vi "popup_timer.vi"(1 "Seconds":dbl) -> (8 "Done":bool)   [LabVIEW 2016]
panel:
  in  "Time Display":bool
  out "Slide":u8(slide) scale=0.0..6.0
  # "Name"
  # "MVC Countdown"
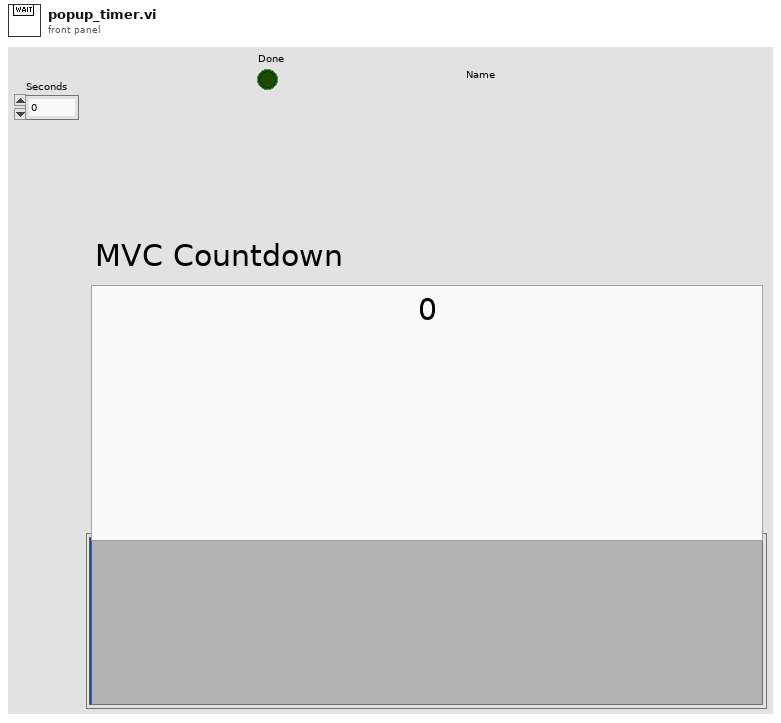
[diagram p1: front panel]
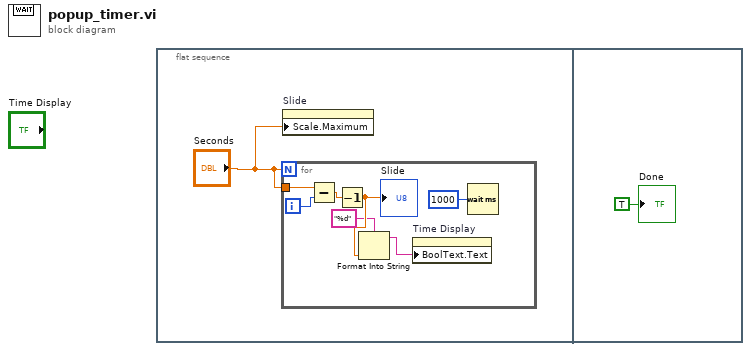
[diagram p0: block diagram]
diagram:
  n1 = flat-sequence {
    frame #0 {
      n2 = for {
        N: "Seconds" -> [_]
        tunnel: "Seconds" -> [w7]
        i -> [w6]
        n3 = Subtract(x=w7, y=w6) -> (x-y=w5:dbl)
        n4 = Decrement(x=w5) -> (x-1=w4:dbl)
        "Slide" <- w4
        n5 = Format Into String(format string="%d", w4) -> (resulting string=w3:string)  [unwired: 2 in, 1 out]
        n6 = property on="Time Display" class="Bool"("BoolText.Text"=w3) -> ()  [unwired: 2 in, 2 out]
        n7 = Wait (ms)(milliseconds to wait=u32 1000) -> ()  [unwired: 1 out]
      }
      n8 = property on="Slide" class="Slide (strict)"("Scale.Maximum"="Seconds") -> ()  [unwired: 2 in, 2 out]
    }
    frame #1 {
      "Done" <- TRUE ("Done")
    }
  }
